vi "MS SQL_Exec_Queury.vi"(8 "error in (no error)":errorcluster, 10 "Query":string, 11 "Refnum in":T1) -> (0 "error out":errorcluster, 1 "Data[]":variant[][](array[variant]), 2 "Data":string[][](array[string]), 3 "Refnum out":T1)   [LabVIEW 2020]
uses:
  <vilib>/addons/database/Connection.llb/Conn ObjectReference.ctl
  <vilib>/addons/database/Connection.llb/Conn Execute.vi
  <vilib>/addons/database/Recordset.llb/Rec Fetch Recordset Data (R).vi
  <vilib>/addons/database/Recordset.llb/Rec Destroy - Connection.vi
  <vilib>/addons/database/NI_Database_API.lvlib
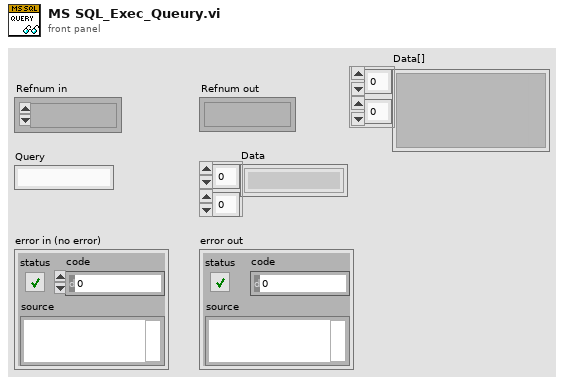
[diagram p1: front panel]
types:
  T1 = typedef "NI_Database_API.lvlib/Conn ObjectReference.ctl" = refnum<k1>
  T2 = typedef "NI_Database_API.lvlib/Rec ObjectReference.ctl" = refnum<k1>
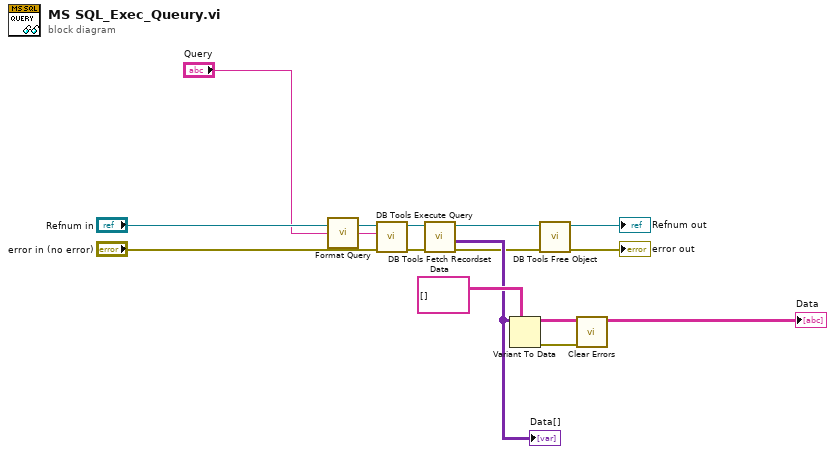
[diagram p0: block diagram]
diagram:
  n1 = call "Format Query.vi"("CMD in"="Query") -> ("CMD out"=w1:string)
  n2 = call-poly <vilib>:"DB Tools Execute Query.vi"("error in (no error)"="error in (no error)", "SQL query"=w1, "connection reference"="Refnum in") -> ("error out"=w5:errorcluster, "recordset reference"=w4:T2)  [unwired: 5 in]
  n3 = call-poly <vilib>:"DB Tools Fetch Recordset Data.vi"("error in (no error)"=w5, "recordset reference"=w4) -> ("error out"=w9:errorcluster, "recordset data"=w11:variant[][], "recordset reference out"=w7:T2)  [unwired: 3 in]
  "Data[]" <- w11
  n4 = Variant To Data(type=string[][] [], Variant=w11) -> (data=→"Data":string[][], error out=w14:errorcluster)  [unwired: 1 in]
  n5 = call-poly <vilib>:"DB Tools Free Object.vi"("error in (no error)"=w9, "recordset reference"=w7) -> ("error out"=→"error out":errorcluster, "connection reference"=→"Refnum out":T1)  [unwired: 8 in]
  n6 = call <vilib>:"Clear Errors.vi"("error in (no error)"=w14) -> ()  [unwired: 5 in, 2 out]
